vi "Heater Control.vi"(8 "error in":errorcluster, 11 "Results in":refnum<class "Cryo Sep Results.lvclass">) -> (0 "error out":errorcluster, 2 "Htr MOS Ctrl":dbl, 3 "Results out":refnum<class "Cryo Sep Results.lvclass">)   [LabVIEW 2019, in "Results.lvlib" / "Cryo Sep Results.lvclass"]
uses:
  Cryo Sep Results.lvclass
  Cryo Sep Results.lvclass/Cryo Sep Results.ctl
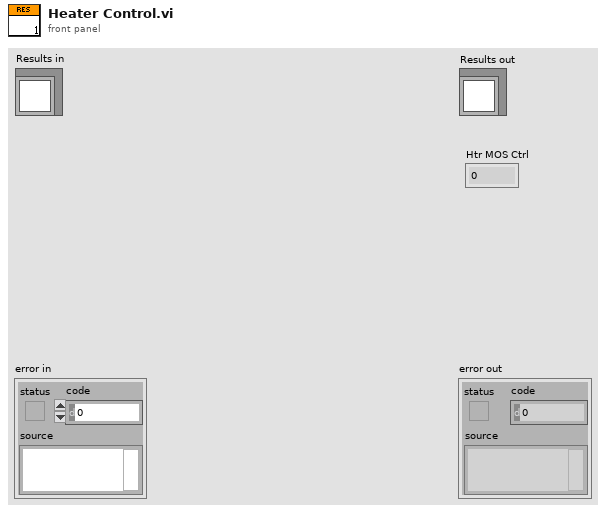
[diagram p1: front panel]
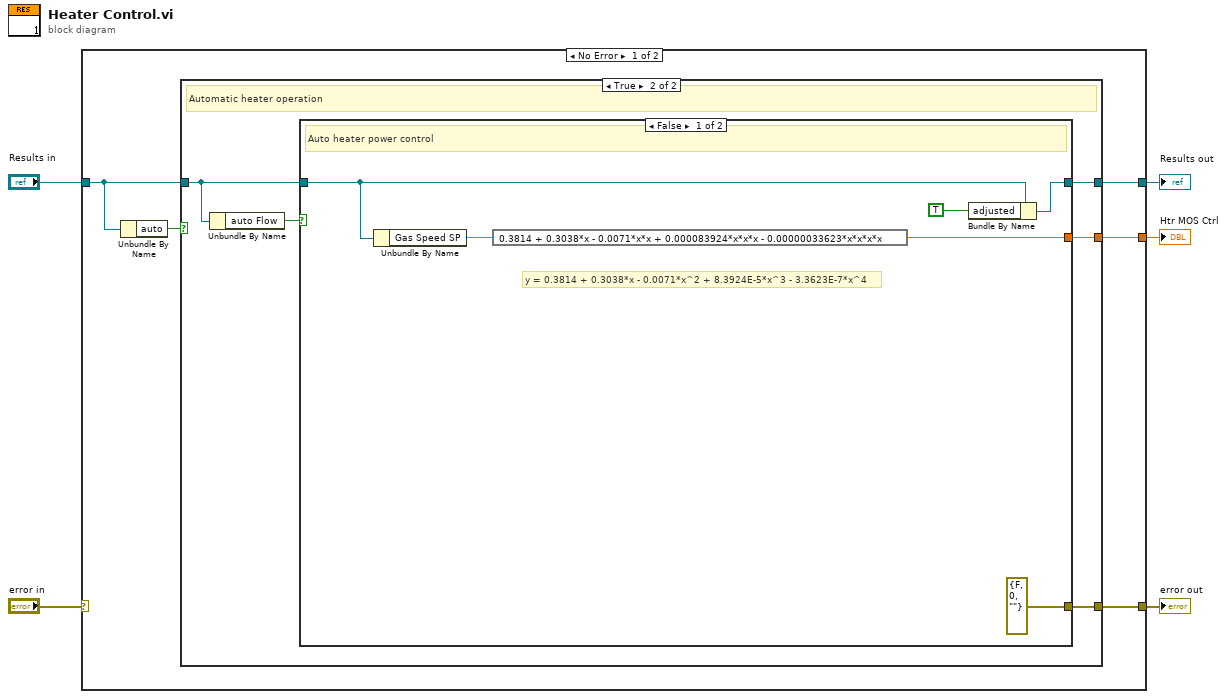
[diagram p0: block diagram]
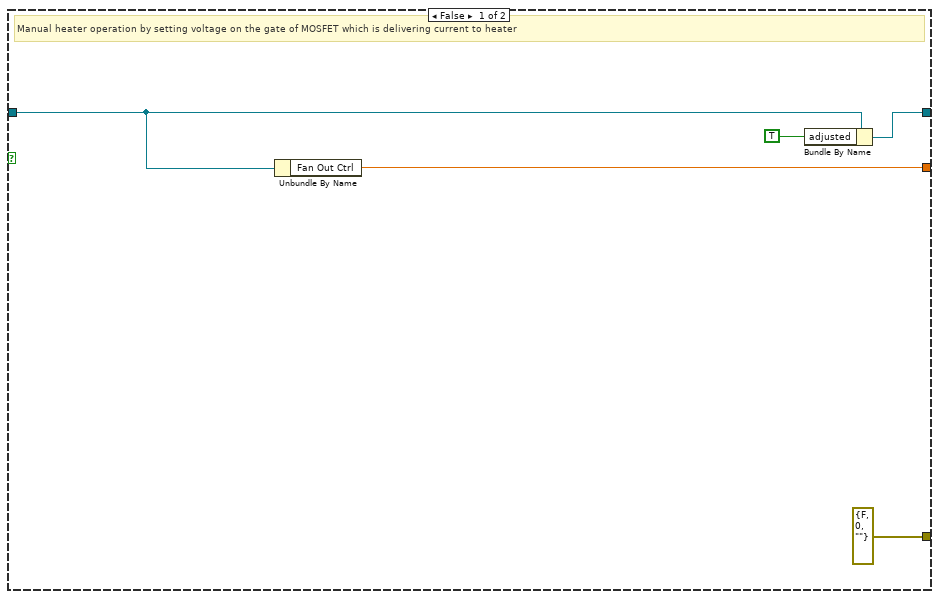
[diagram p2: hidden frame]
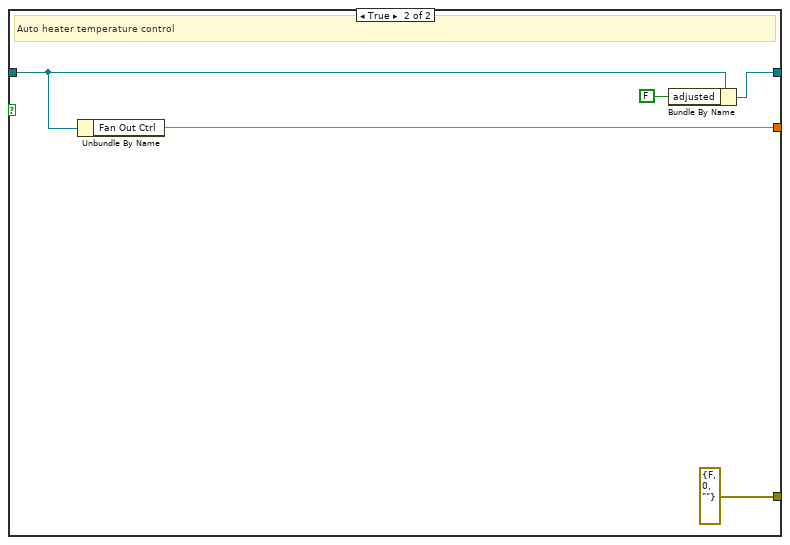
[diagram p3: hidden frame]
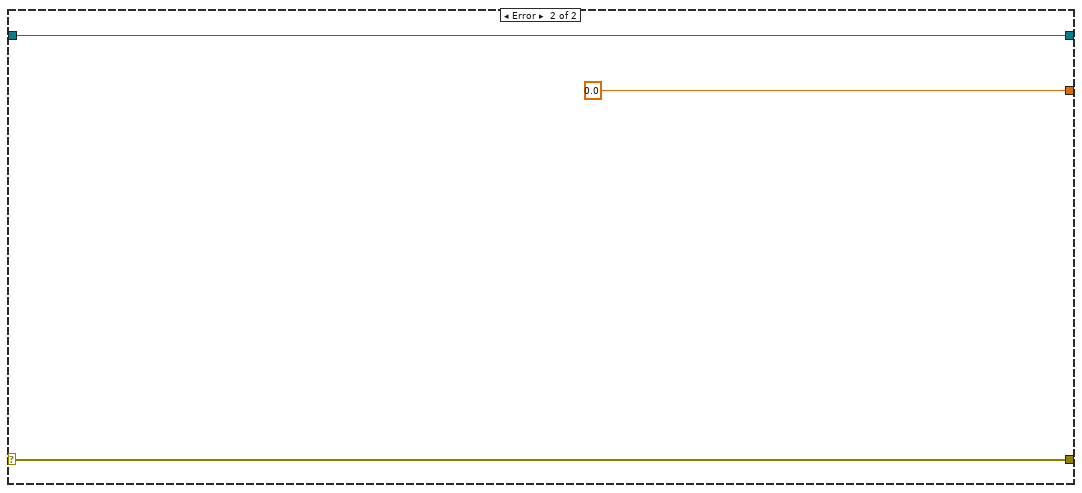
[diagram p4: hidden frame]
diagram:
  n1 = case shown="No Error" "error in" {
    selector: "error in" -> [_ w34]
    tunnel: [w7 w34] -> w4
    tunnel: "Results in" -> [w9 w32]
    tunnel: [w10 0.0 ("Htr MOS Ctrl")] -> w2
    tunnel: [w6 w32] -> w1
    frame No Error {
      n2 = Unbundle By Name(w9) -> ("auto"=w8:bool)
      n3 = case shown="True" w8 {
        tunnel: [w15 w18] -> w10
        tunnel: w9 -> [w13 w20]
        tunnel: [errorcluster {"status"=FALSE, "code"=0, "source"=""} ("error IO") w17] -> w7
        tunnel: [w11 w16] -> w6
        frame False {
          # "Manual heater operation by setting voltage on the gate of MOSFET which is delivering current to heater"
          n4 = Unbundle By Name(w13) -> ("Fan Out Ctrl"=w15:dbl)
          n5 = Bundle By Name(cluster=w13, "adjusted"=TRUE) -> (w11:refnum<class "Cryo Sep Results.lvclass">)
        }
        frame True {
          # "Automatic heater operation"
          n6 = Unbundle By Name(w20) -> ("auto Flow"=w19:bool)
          n7 = case shown="False" w19 {
            tunnel: w20 -> [w23 w29]
            tunnel: [w21 w31] -> w18
            tunnel: [errorcluster {"status"=FALSE, "code"=0, "source"=""} ("error IO") errorcluster {"status"=FALSE, "code"=0, "source"=""} ("error IO")] -> w17
            tunnel: [w25 w28] -> w16
            frame False {
              # "y = 0.3814 + 0.3038*x - 0.0071*x^2 + 8.3924E-5*x^3 - 3.3623E-7*x^4"
              # "Auto heater power control"
              n8 = Unbundle By Name(w23) -> ("Gas Speed SP"=w22:dbl)
              n9 = expression code="0.3814 + 0.3038*x - 0.0071*x*x + 0.000083924*x*x*x - 0.00000033623*x*x*x*x"(w22) -> (w21:dbl)
              n10 = Bundle By Name(cluster=w23, "adjusted"=TRUE) -> (w25:refnum<class "Cryo Sep Results.lvclass">)
            }
            frame True {
              # "Auto heater temperature control"
              n11 = Unbundle By Name(w29) -> ("Fan Out Ctrl"=w31:dbl)
              n12 = Bundle By Name(cluster=w29, "adjusted"=FALSE) -> (w28:refnum<class "Cryo Sep Results.lvclass">)
            }
          }
        }
      }
    }
    frame Error {
    }
  }
  "error out" <- w4
  "Htr MOS Ctrl" <- w2
  "Results out" <- w1
